vi "UVI_PopUp Menu_Item_Track.vi"(0 "hMenu":u32, 5 "Menu params":T1, 7 "Mouse position":cluster{"x":i32, "y":i32}, 9 "Active Window handle":u32, 11 "error in (no error)":errorcluster) -> (8 "MenuSelection":u32, 15 "error out":errorcluster)   [LabVIEW 2013]
uses:
  TD_PopUp Menu_Parameters.ctl
  user32.dll
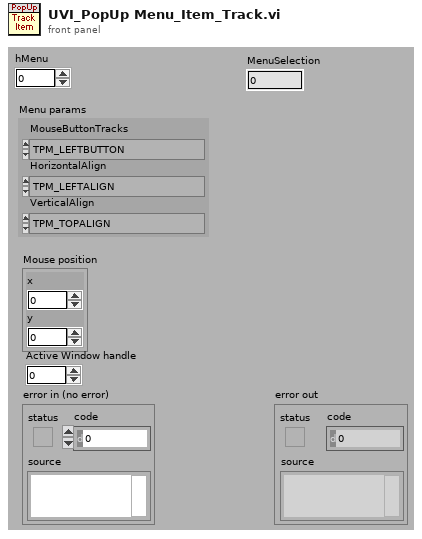
[diagram p1: front panel]
types:
  T1 = typedef "TD_PopUp Menu_Parameters.ctl" = cluster{"MouseButtonTracks":enum16{"TPM_LEFTBUTTON", "TPM_RIGHTBUTTON"}, "HorizontalAlign":enum16{"TPM_LEFTALIGN", "TPM_CENTRALALIGN", "TPM_RIGHTALIGN"}, "VerticalAlign":enum16{"TPM_TOPALIGN", "TPM_CENTRALALIGN", "TPM_BOTTOMALIGN"}}
  T2 = enum16{"TPM_LEFTALIGN", "TPM_CENTRALALIGN", "TPM_RIGHTALIGN"}
  T3 = enum16{"TPM_TOPALIGN", "TPM_CENTRALALIGN", "TPM_BOTTOMALIGN"}
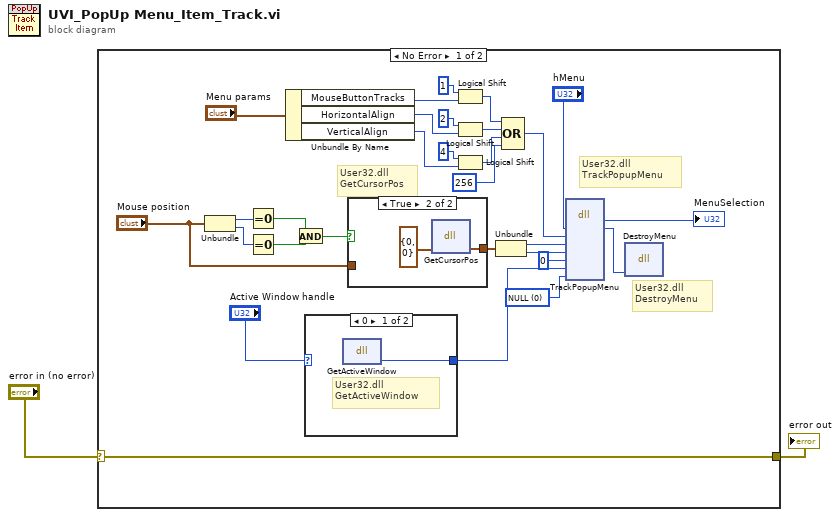
[diagram p0: block diagram]
diagram:
  n1 = case shown="No Error" "error in (no error)" {
    selector: "error in (no error)" -> [w3 w37]
    tunnel: [w3 w37] -> w1
    frame No Error {
      w14 = u16 0 items=["NULL"]
      # "User32.dll\nDestroyMenu"
      # "User32.dll\nTrackPopupMenu"
      # "User32.dll\nGetCursorPos"
      n2 = Unbundle("Mouse position") -> ("x"=w26:i32, "y"=w27:i32)
      n3 = Equal To 0?(x=w26) -> (x = 0?=w28:bool)
      n4 = Equal To 0?(x=w27) -> (x = 0?=w29:bool)
      n5 = Unbundle By Name("Menu params") -> ("MouseButtonTracks"=w21:enum16{"TPM_LEFTBUTTON", "TPM_RIGHTBUTTON"}, "HorizontalAlign"=w22:T2, "VerticalAlign"=w23:T3)
      n6 = And(x=w28, y=w29) -> (x .and. y?=w30:bool)
      n7 = case shown="0" "Active Window handle" {
        selector: "Active Window handle" -> [_ w36]
        tunnel: [w35 w36] -> w15
        frame 0 {
          # "User32.dll\nGetActiveWindow"
          n8 = dll-call lib="User32" fn="GetActiveWindow"() -> (w35:u32)  [unwired: 3 in, 2 out]
        }
        frame 1, Default {
        }
      }
      n9 = case shown="True" w30 {
        tunnel: [w32 w34] -> w25
        tunnel: "Mouse position" -> [w32 _]
        frame False {
        }
        frame True {
          n10 = dll-call lib="user32.dll" fn="GetCursorPos"("Mouse position"=cluster{"x":i32, "y":i32} {"x"=0, "y"=0}) -> ("Mouse position"=w34:cluster{"x":i32, "y":i32})  [unwired: 3 in, 3 out]
        }
      }
      n11 = Logical Shift(y=1, x=w21) -> (x << y=w8:u32)
      n12 = Logical Shift(y=2, x=w22) -> (x << y=w9:u32)
      n13 = Logical Shift(y=4, x=w23) -> (x << y=w10:u32)
      n14 = Unbundle(w25) -> ("x"=w13:i32, "y"=w12:i32)
      n15 = Compound Arithmetic op=OR(w8, w9, w10, u32 256) -> (w11:u32)
      n16 = dll-call lib="user32.dll" fn="TrackPopupMenu"("hMenu"="hMenu", "uFlags"=w11, "x"=w13, "y"=w12, "nReserved"=0, "hwnd"=w15, w14) -> ("bool"=→"MenuSelection":u32, "hMenu"=w24:u32)  [unwired: 8 in, 3 out]
      n17 = dll-call lib="User32" fn="DestroyMenu"("hMenu"=w24) -> ()  [unwired: 4 in, 3 out]
    }
    frame Error {
    }
  }
  "error out" <- w1
